vi "PathPlanner_GridPosition_Equals.vi"(9 "Other GridPosition":T1, 11 "GridPosition":T1) -> (3 "Equal":bool)   [LabVIEW 2019, in "PathPlanner24.lvlib"]
uses:
  PathPlanner24.lvlib
  TypeDef/PathPlannerFinderGridPosition.ctl
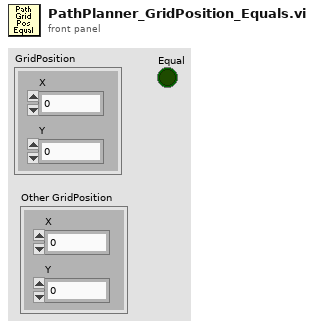
[diagram p1: front panel]
types:
  T1 = typedef "PathPlanner24.lvlib/PathPlannerFinderGridPosition.ctl" = cluster{"X":i32, "Y":i32}
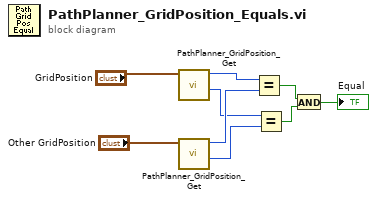
[diagram p0: block diagram]
diagram:
  n1 = call "PathPlanner_GridPosition_Get.vi"("GridPosition"="GridPosition") -> ("Int Y"=w5:i32, "Int X"=w7:i32)  [unwired: 9 in]
  n2 = call "PathPlanner_GridPosition_Get.vi"("GridPosition"="Other GridPosition") -> ("Int Y"=w4:i32, "Int X"=w6:i32)  [unwired: 9 in]
  n3 = Equal?(x=w7, y=w6) -> (x = y?=w3:bool)
  n4 = Equal?(x=w5, y=w4) -> (x = y?=w2:bool)
  n5 = And(x=w3, y=w2) -> (x .and. y?=→"Equal":bool)
